vi "Check Threads For State.vi"(8 "error in (no error)":errorcluster, 10 "state":T1, 11 "Framework in":refnum<class "Framework.lvclass">) -> (0 "error out":errorcluster, 1 "private threads equal":bool[](array[boolean]), 2 "public threads equal":bool[](array[boolean]), 3 "Framework out":refnum<class "Framework.lvclass">)   [LabVIEW 2019, in "DSF Core.lvlib" / "Framework.lvclass"]
uses:
  Framework.lvclass
  Thread/Thread State.ctl
  Thread/Thread.lvclass
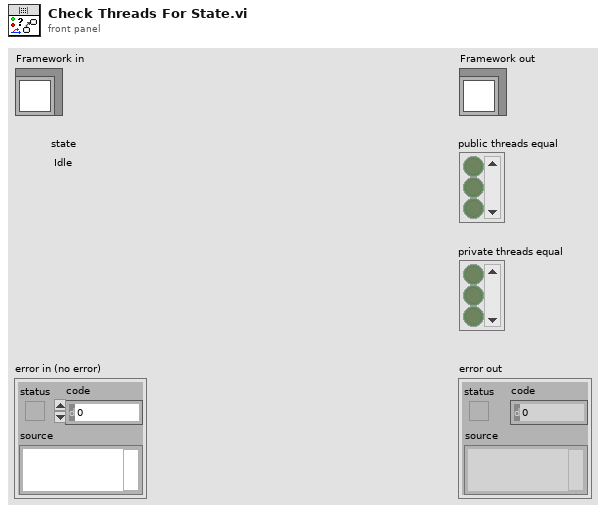
[diagram p1: front panel]
types:
  T1 = typedef "DSF Core.lvlib/Thread.lvclass/Thread State.ctl" = enum8{"Idle", "Running", "Error", "Shut Down"}
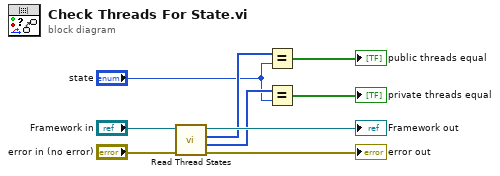
[diagram p0: block diagram]
diagram:
  n1 = call "Read Thread States.vi"("error in (no error)"="error in (no error)", "Framework in"="Framework in") -> ("error out"=→"error out":errorcluster, "private thread states"=w5:T1[], "public thread states"=w4:T1[], "Framework out"=→"Framework out":refnum<class "Framework.lvclass">)  [unwired: 6 in]
  n2 = Equal?(x=w4, y="state") -> (x = y?=→"public threads equal":bool[])
  n3 = Equal?(x=w5, y="state") -> (x = y?=→"private threads equal":bool[])
